vi "Tek_Set.vi"(8 "error in (no error)":errorcluster, 9 "range":T1, 10 "Scope":cluster{dbl, dbl, dbl[]}(graph), 11 "plot":refnum<vi>) -> ()   [LabVIEW 2022 SP3]
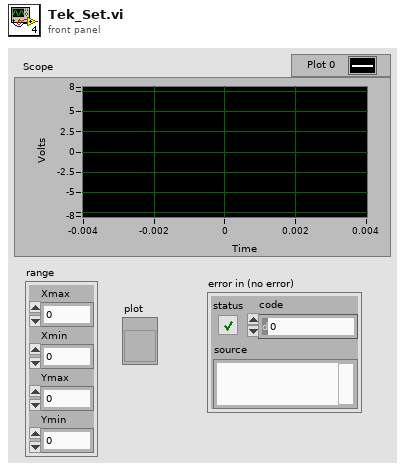
[diagram p1: front panel]
types:
  T1 = cluster{"Xmax":dbl, "Xmin":dbl, "Ymax":dbl, "Ymin":dbl}
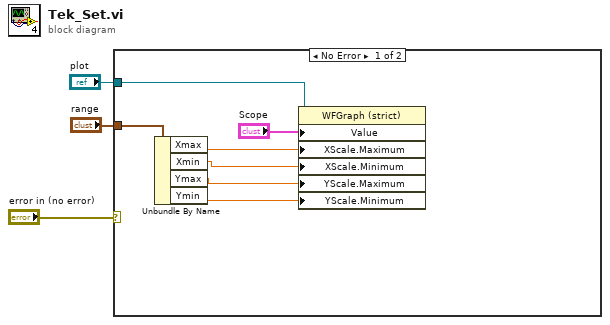
[diagram p0: block diagram]
diagram:
  n1 = case shown="No Error" "error in (no error)" {
    tunnel: "range" -> [w10 _]
    tunnel: "plot" -> [w4 _]
    frame No Error {
      n2 = Unbundle By Name(w10) -> ("Xmax"=w9:dbl, "Xmin"=w8:dbl, "Ymax"=w7:dbl, "Ymin"=w6:dbl)
      n3 = property class="WFGraph (strict)"(reference=w4, "Value"="Scope", "XScale.Maximum"=w9, "XScale.Minimum"=w8, "YScale.Maximum"=w7, "YScale.Minimum"=w6) -> ()  [unwired: 1 in, 2 out]
    }
    frame Error {
    }
  }
